vi "fps.vi"() -> (0 "FPS":dbl format="%#.1f")   [LabVIEW 2010]
doc: "Averages over 30 iterations the speed of a loop structure.\n<B>FPS</B> represents Frames (iterations) per Second."
panel:
  in  "Array":u32[](array[numeric])=[0, 0, 0, 0, 0, 0, 0, 0, 0, 0, 0, 0, 0, 0, 0, 0, 0, 0, 0, 0, 0, 0, 0, 0, 0, 0, 0, 0, 0, 0]
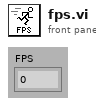
[diagram p1: front panel]
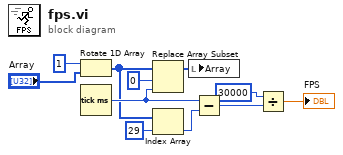
[diagram p0: block diagram]
diagram:
  n1 = Rotate 1D Array(1:"Array", 2:1 ("n")) -> (0:w5:u32[])
  n2 = Tick Count (ms)() -> (millisecond timer value=w7:u32)
  n3 = Replace Array Subset(array=w5, new element=w7, index=0) -> (w8:u32[])
  n4 = Index Array(array=w5, index=29) -> (element=w6:u32)
  n5 = local write "Array"(w8) -> ()
  n6 = Subtract(x=w7, y=w6) -> (x-y=w9:u32)
  n7 = Divide(x=u32 30000, y=w9) -> (x/y=→"FPS":dbl)
